vi "Step UI Main.vi"(8 "error in (no error)":errorcluster, 11 "Step UI in":refnum<class "Step UI.lvclass">) -> (0 "error out":errorcluster, 3 "Step UI out":refnum<class "Step UI.lvclass">)   [LabVIEW 2015, in "Step UI.lvclass"]
uses:
  Step UI.lvclass
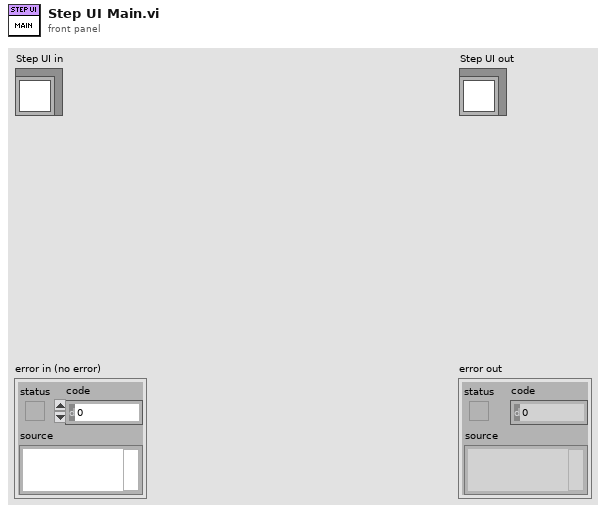
[diagram p1: front panel]
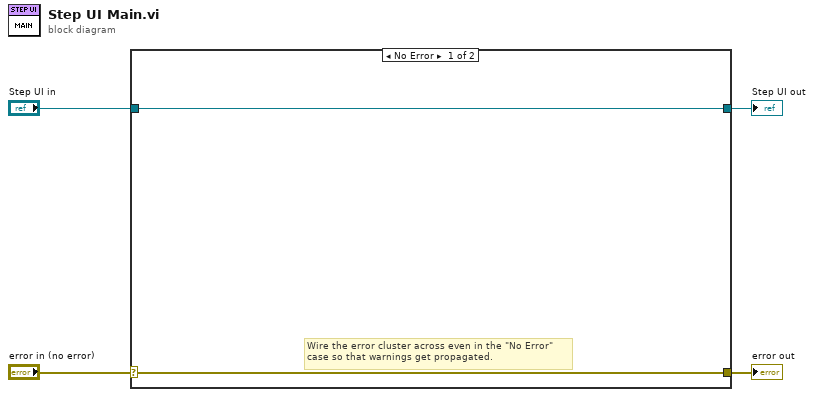
[diagram p0: block diagram]
diagram:
  n1 = case shown="No Error" "error in (no error)" {
    selector: "error in (no error)" -> [w5 w8]
    tunnel: [w5 w8] -> w3
    tunnel: [w6 w7] -> w1
    tunnel: "Step UI in" -> [w6 w7]
    frame No Error {
      # "Wire the error cluster across even in the \"No Error\"\ncase so that warnings get propagated."
    }
    frame Error {
    }
  }
  "error out" <- w3
  "Step UI out" <- w1
